vi "StateElevator.vi"(0 "Master State In":T1(ring)) -> ()   [LabVIEW 2023]
doc: "This VI performs all of the calculations and decisions related to the swerve drive."
uses:
  da1023b0-1576-4aac-9f1b-c0fc6dfe0547.vi
  a50a7afd-ca11-4ff6-935c-5d6bedee04cc.vi
  GlobalElevator.vi
  GlobalDriverStationCommands.vi
panel:
  in  "Trap Elevator Position (in)":dbl
  in  "Elevator acceptable error (in)":dbl=0.5
  in  "Climbing outer position (in)":dbl=21.0
  in  "Amp Elevator Position (in)":dbl=7.0
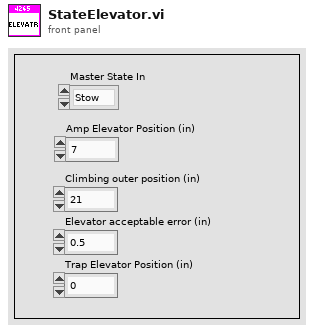
[diagram p1: front panel]
types:
  T1 = enum16{"Stow", "Speaker", "Amp", "Climbing", "Trap"}
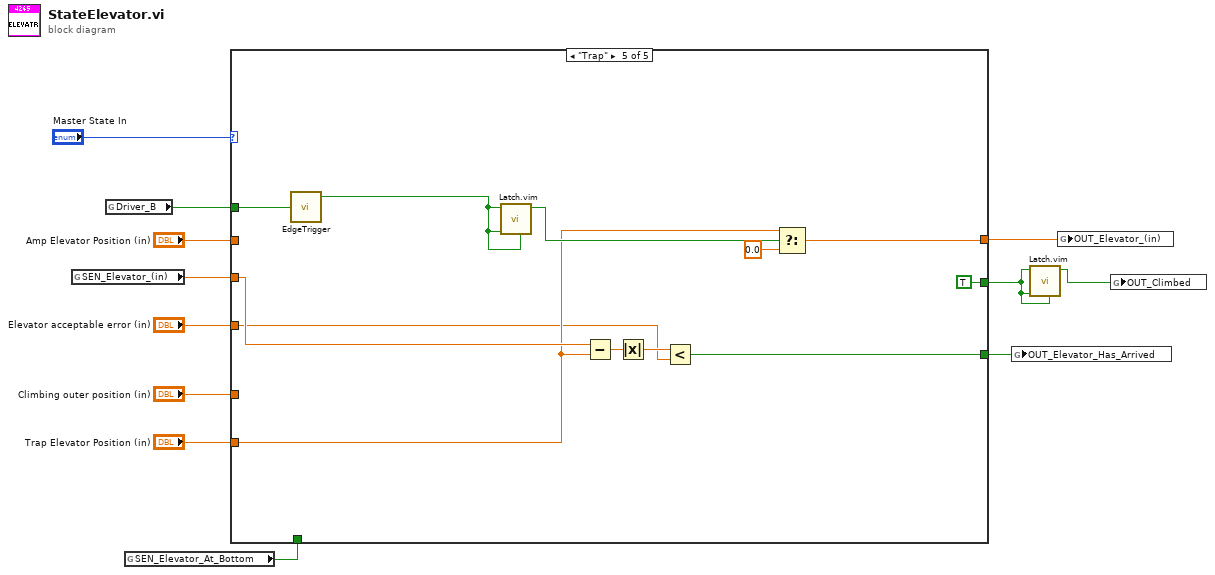
[diagram p0: block diagram]
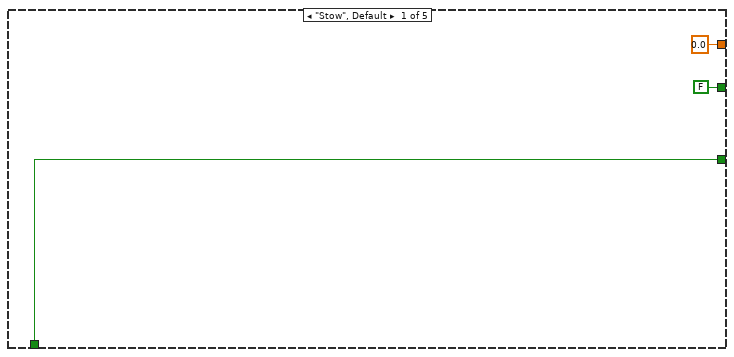
[diagram p2: hidden frame]
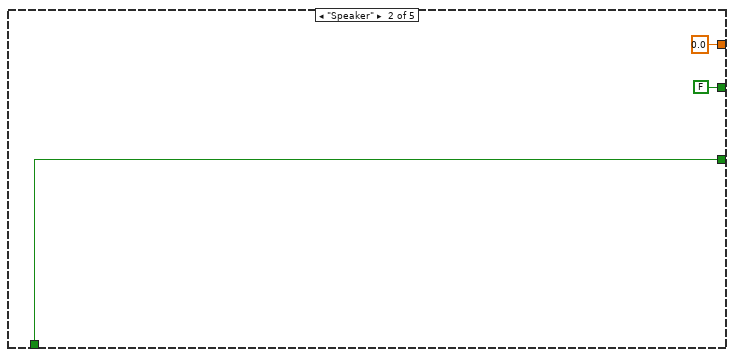
[diagram p3: hidden frame]
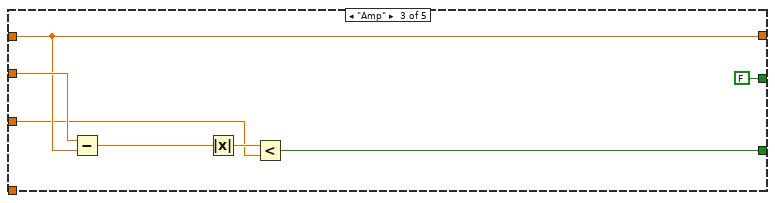
[diagram p4: hidden frame]
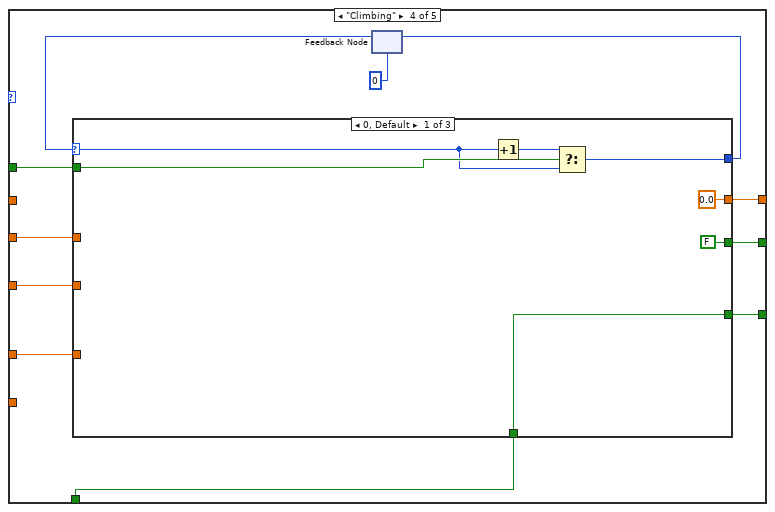
[diagram p5: hidden frame]
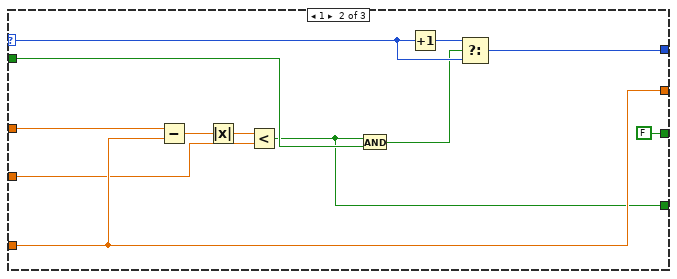
[diagram p6: hidden frame]
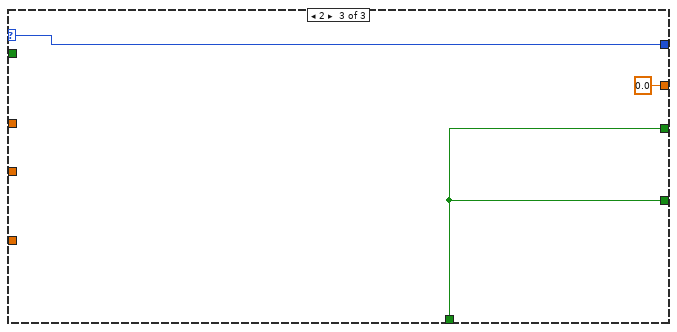
[diagram p7: hidden frame]
diagram:
  n1 = global read "GlobalElevator.vi" "SEN_Elevator_(in)"() -> (w4:dbl)
  n2 = global read "GlobalDriverStationCommands.vi" "Driver_B"() -> (w6:bool)
  n3 = global read "GlobalElevator.vi" "SEN_Elevator_At_Bottom"() -> (w2:bool)
  n4 = case shown="\"Trap\"" "Master State In" {
    tunnel: [0.0 ("f") 0.0 ("f") w22 w32 w69] -> w12
    tunnel: "Amp Elevator Position (in)" -> [_ _ w22 _ _]
    tunnel: w4 -> [_ _ w23 w31 w65]
    tunnel: "Climbing outer position (in)" -> [_ _ _ w33 _]
    tunnel: "Elevator acceptable error (in)" -> [_ _ w20 w30 w63]
    tunnel: [FALSE ("SEN_Elevator_At_Bottom") FALSE FALSE w29 TRUE] -> w8
    tunnel: "Trap Elevator Position (in)" -> [_ _ _ _ w64]
    tunnel: w6 -> [_ _ _ w28 w60]
    tunnel: [w15 w17 w19 w27 w61] -> w5
    tunnel: w2 -> [w15 w17 _ w26 _]
    frame "Stow", Default {
    }
    frame "Speaker" {
    }
    frame "Amp" {
      n5 = Subtract(x=w23, y=w22) -> (x-y=w21:dbl)
      n6 = Absolute Value(x=w21) -> (abs(x)=w24:dbl)
      n7 = Less?(x=w24, y=w20) -> (x < y?=w19:bool)
    }
    frame "Climbing" {
      n8 = feedback #1(0) -> (w35:i32)
      n9 = case shown="0, Default" w35 {
        selector: w35 -> [w40 w48 w57]
        tunnel: [w43 w55 w57] -> w34
        tunnel: w33 -> [_ w53 _]
        tunnel: [0.0 ("Climbing outer position") w53 0.0 ("Climbing outer position")] -> w32
        tunnel: w31 -> [_ w54 _]
        tunnel: w30 -> [_ w52 _]
        tunnel: [FALSE ("SEN_Elevator_At_Bottom") FALSE w56] -> w29
        tunnel: w28 -> [w42 w46 _]
        tunnel: [w39 w44 w56] -> w27
        tunnel: w26 -> [w39 _ w56]
        frame 0, Default {
          n10 = Increment(x=w40) -> (x+1=w41:i32)
          n11 = Select(t=w41, s=w42, f=w40) -> (s? t:f=w43:i32)
        }
        frame 1 {
          n12 = Subtract(x=w54, y=w53) -> (x-y=w51:dbl)
          n13 = Absolute Value(x=w51) -> (abs(x)=w50:dbl)
          n14 = Less?(x=w50, y=w52) -> (x < y?=w44:bool)
          n15 = And(x=w44, y=w46) -> (x .and. y?=w45:bool)
          n16 = Increment(x=w48) -> (x+1=w49:i32)
          n17 = Select(t=w49, s=w45, f=w48) -> (s? t:f=w55:i32)
        }
        frame 2 {
        }
      }
      n18 = feedback-in #1(w34) -> ()
    }
    frame "Trap" {
      n19 = call "EdgeTrigger.vi"("Input Signal"=w60) -> ("Rising Edge Trigger"=w59:bool)  [unwired: 2 out]
      n20 = call "Latch.vim"("Default Value"=w59, "Latch Signal"=w59, "Latch Value"=w59) -> ("Latched"=w68:bool)  [unwired: 8 in]
      n21 = Subtract(x=w65, y=w64) -> (x-y=w62:dbl)
      n22 = Absolute Value(x=w62) -> (abs(x)=w66:dbl)
      n23 = Less?(x=w66, y=w63) -> (x < y?=w61:bool)
      n24 = Select(t=w64, s=w68, f=0.0) -> (s? t:f=w69:dbl)
    }
  }
  n25 = global write "GlobalElevator.vi" "OUT_Elevator_Has_Arrived"(w5) -> ()
  n26 = call "Latch.vim"("Default Value"=w8, "Latch Signal"=w8, "Latch Value"=w8) -> ("Latched"=w7:bool)  [unwired: 8 in]
  n27 = global write "GlobalElevator.vi" "OUT_Elevator_(in)"(w12) -> ()
  n28 = global write "GlobalElevator.vi" "OUT_Climbed"(w7) -> ()
